vi "SetParam.vi"(8 "error in (no error)":errorcluster caption="entrée d'erreur (pas d'erreur)", 10 "average_precision_score":T1={"average"="macro", "pos_label"={"dtype_pos_label"="int", "pos_label"="1"}, "sample_weight"=[]}, 11 "Average_Precision_Score.lvclass":refnum<class "Average_Precision_Score.lvclass">) -> (0 "error out":errorcluster caption="sortie d'erreur", 3 "Average_Precision_Score.lvclass":refnum<class "Average_Precision_Score.lvclass">)   [LabVIEW 2020, in "Average_Precision_Score.lvclass"]
doc: "Set Parameters"
uses:
  Average_Precision_Score.lvclass
  Average_Precision_Score.lvclass/Average_Precision_Score.ctl
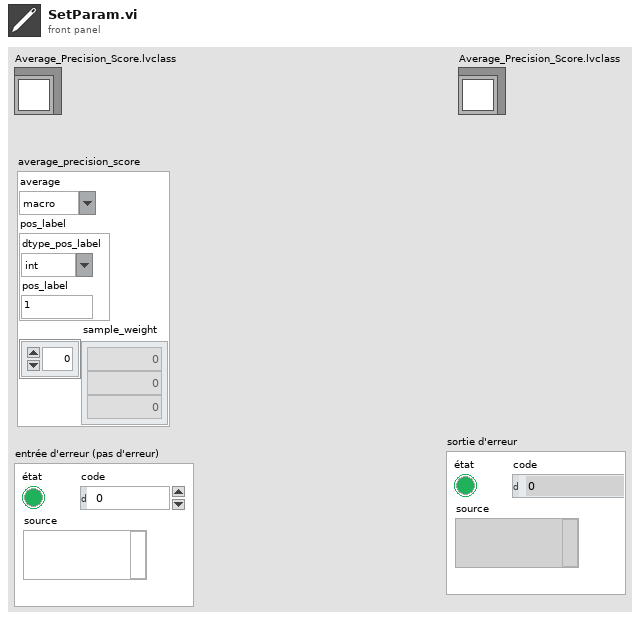
[diagram p1: front panel]
types:
  T1 = cluster{"average":string, "pos_label":cluster{"dtype_pos_label":string, "pos_label":string}, "sample_weight":dbl[]}
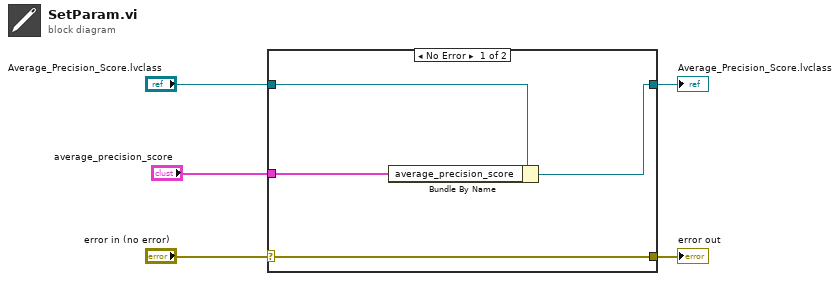
[diagram p0: block diagram]
diagram:
  n1 = case shown="No Error" "error in (no error)" {
    selector: "error in (no error)" -> [w9 w10]
    tunnel: [w9 w10] -> w4
    tunnel: [w7 w11] -> w2
    tunnel: "Average_Precision_Score.lvclass" -> [w8 w11]
    tunnel: "average_precision_score" -> [w6 _]
    frame No Error {
      n2 = Bundle By Name(cluster=w8, "average_precision_score"=w6) -> (w7:refnum<class "Average_Precision_Score.lvclass">)
    }
    frame Error {
    }
  }
  "error out" <- w4
  "Average_Precision_Score.lvclass" <- w2
